vi "ExpressionNodeNotesMarcoGonzalez.vi"() -> ()   [LabVIEW 2012]
panel:
  out "Numeric 2":dbl
  in  "Numeric":dbl
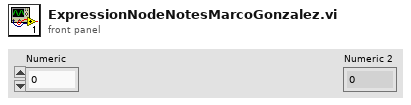
[diagram p1: front panel]
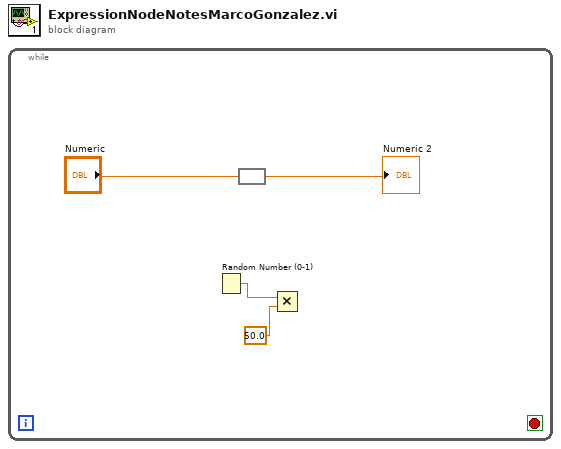
[diagram p0: block diagram]
diagram:
  n1 = while {
    stop <- _ stop-if-true
    n2 = Random Number (0-1)() -> (number: 0 to 1=w4:dbl)
    n3 = expression code=""("Numeric") -> (→"Numeric 2":dbl)
    n4 = Multiply(x=w4, y=50.0) -> ()  [unwired: 1 out]
  }
